vi "Quadrature-Input.vi"() -> ()   [LabVIEW 2020]
panel:
  out "Direction":string
  out "Error String":string
  out "error out":errorcluster
  in  "error in (no error)":errorcluster
  out "ConnectionType Out":i32
  out "DeviceType Out":i32
  in  "Identifier":string="LJM_idANY"
  in  "Connection Type":string="LJM_ctANY"
  in  "Device Type":string="LJM_dtANY"
  out "Revolutions":i32
  in  "?":bool
  in  "Phase Pairs":T1(ring)=enum."T7/T4: FIO6 + FIO7"
  in  "Encoder counts per revolution":i32=400
  in  "stop":bool
  out "Guage":dbl(knob) min=0.0 max=360.0 step=15.0 scale=0.0..360.0
  out "Degrees From Zero":i32
  out "Enc 2's Comp":dbl
  out "Enc Float":dbl
  # "T4 Capable DIO: DIO4, DIO5, DIO6, DIO7, DIO8, DIO9 (aka FIO4, FIO5, FIO6, FIO7, EIO0, EIO1)\n \nT7 Capable DIO: DIO0, DIO1, DIO2, DIO3, DIO6, DIO7 (aka FIO0, FIO1, FIO2, FIO3, FIO6, FIO7)\n\nThe channels must be used in one of the consecutive pairs that can be selected below in \"Phase Pairs\" .The even channel is Phase A and odd channel is Phase B of the encoder.\n\nMake sure to set how many counts per revolution for the encoder."
  # "0"
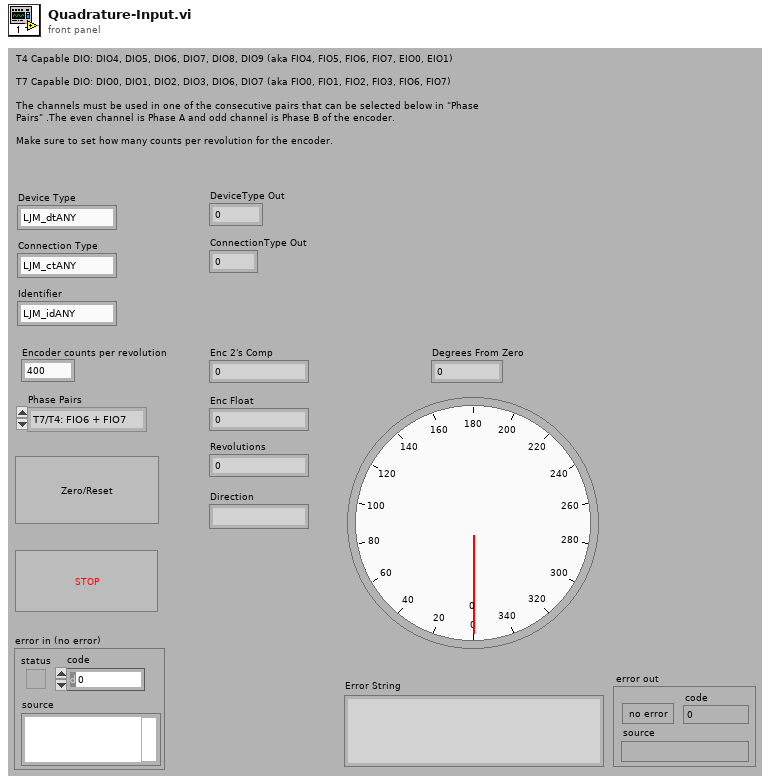
[diagram p1: front panel]
types:
  T1 = enum16{"T7: FIO0 + FIO1", "T7: FIO2 + FIO3", "T7/T4: FIO6 + FIO7", "T4: FIO4 + FIO5", "T4: EIO0 + EIO1"}
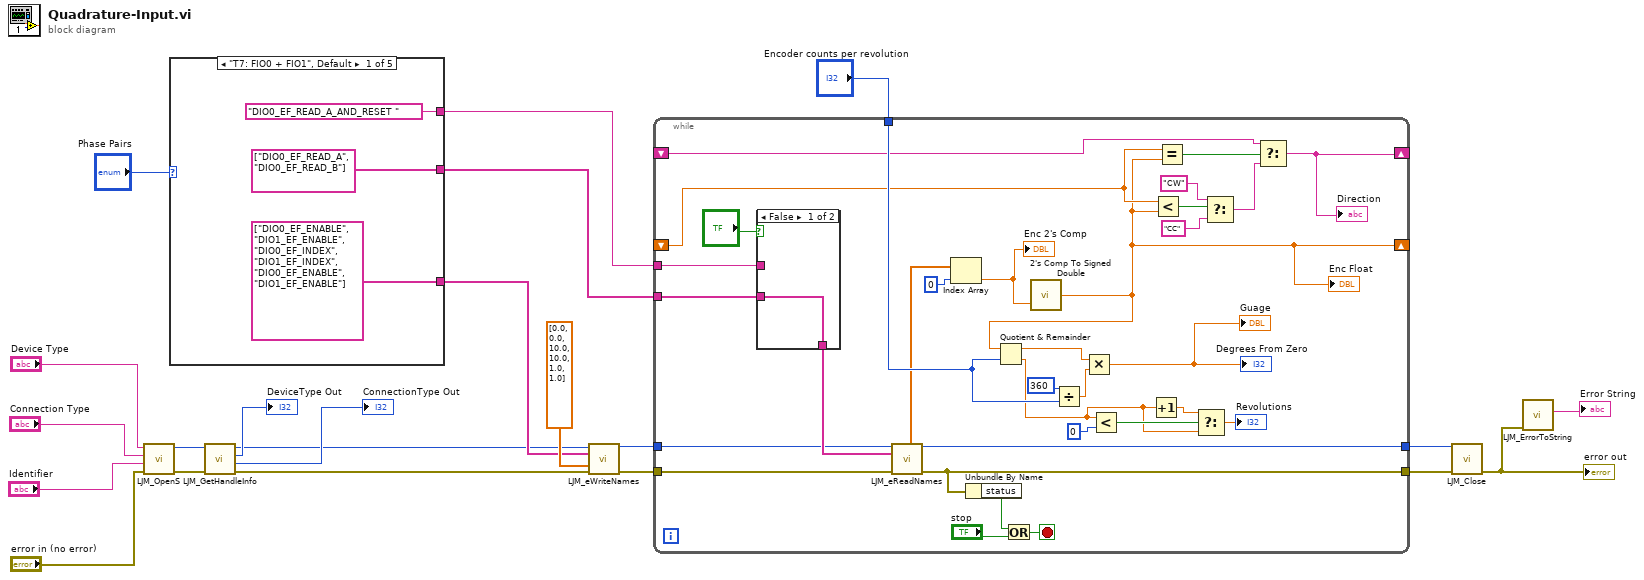
[diagram p0: block diagram]
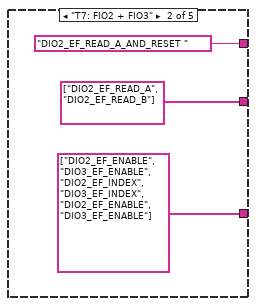
[diagram p2: hidden frame]
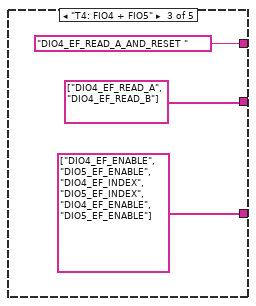
[diagram p3: hidden frame]
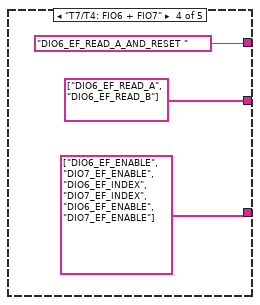
[diagram p4: hidden frame]
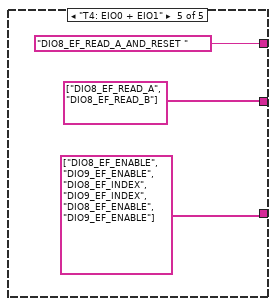
[diagram p5: hidden frame]
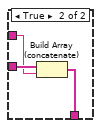
[diagram p6: hidden frame]
diagram:
  n1 = call "LJM_OpenS.vi"("error in"="error in (no error)", "Identifier"="Identifier", "ConnectionType"="Connection Type", "DeviceType"="Device Type") -> ("error out"=w21:errorcluster, "Handle"=w20:i32)  [unwired: 6 in]
  n2 = case shown="\"T7: FIO0 + FIO1\", Default" "Phase Pairs" {
    tunnel: [string[] ["DIO0_EF_READ_A", "DIO0_EF_READ_B"] string[] ["DIO2_EF_READ_A", "DIO2_EF_READ_B"] string[] ["DIO4_EF_READ_A", "DIO4_EF_READ_B"] string[] ["DIO6_EF_READ_A", "DIO6_EF_READ_B"] string[] ["DIO8_EF_READ_A", "DIO8_EF_READ_B"]] -> w9
    tunnel: [string[] ["DIO0_EF_ENABLE", "DIO1_EF_ENABLE", "DIO0_EF_INDEX", "DIO1_EF_INDEX", "DIO0_EF_ENABLE", "DIO1_EF_ENABLE"] string[] ["DIO2_EF_ENABLE", "DIO3_EF_ENABLE", "DIO2_EF_INDEX", "DIO3_EF_INDEX", "DIO2_EF_ENABLE", "DIO3_EF_ENABLE"] string[] ["DIO4_EF_ENABLE", "DIO5_EF_ENABLE", "DIO4_EF_INDEX", "DIO5_EF_INDEX", "DIO4_EF_ENABLE", "DIO5_EF_ENABLE"] string[] ["DIO6_EF_ENABLE", "DIO7_EF_ENABLE", "DIO6_EF_INDEX", "DIO7_EF_INDEX", "DIO6_EF_ENABLE", "DIO7_EF_ENABLE"] string[] ["DIO8_EF_ENABLE", "DIO9_EF_ENABLE", "DIO8_EF_INDEX", "DIO9_EF_INDEX", "DIO8_EF_ENABLE", "DIO9_EF_ENABLE"]] -> w10
    tunnel: ["DIO0_EF_READ_A_AND_RESET " "DIO2_EF_READ_A_AND_RESET " "DIO4_EF_READ_A_AND_RESET " "DIO6_EF_READ_A_AND_RESET " "DIO8_EF_READ_A_AND_RESET "] -> w8
    frame "T7: FIO0 + FIO1", Default {
    }
    frame "T7: FIO2 + FIO3" {
    }
    frame "T4: FIO4 + FIO5" {
    }
    frame "T7/T4: FIO6 + FIO7" {
    }
    frame "T4: EIO0 + EIO1" {
    }
  }
  n3 = call "LJM_GetHandleInfo.vi"("error in"=w21, "Handle In"=w20) -> ("error out"=w13:errorcluster, "ConnectionType"=→"ConnectionType Out":i32, "DeviceType"=→"DeviceType Out":i32, "Handle Out"=w1:i32)  [unwired: 2 in, 4 out]
  n4 = call "LJM_eWriteNames.vi"("Handle In"=w1, "aNames"=w10, "aValuesIn"=dbl[] [0.0, 0.0, 10.0, 10.0, 1.0, 1.0], "error in"=w13) -> ("Handle Out"=w19:i32, "error out"=w18:errorcluster)  [unwired: 9 in, 1 out]
  n5 = while {
    tunnel: w18 -> [w46]
    tunnel: [w67] -> w2
    tunnel: w19 -> [w47]
    tunnel: [w66] -> w3
    tunnel: "Encoder counts per revolution" -> [w64]
    tunnel: w9 -> [w59]
    tunnel: w8 -> [w60]
    shift-right: [w44] -> _
    shift-left: _ -> [w54]
    shift-right: [w49] -> _
    shift-left: _ -> [w50]
    stop <- w70 stop-if-true
    n6 = case shown="False" "?" {
      tunnel: w60 -> [_ w73]
      tunnel: w59 -> [w71 w74]
      tunnel: [w71 w72] -> w58
      frame False {
      }
      frame True {
        n7 = Build Array (concatenate)(w74, w73) -> (w72:string[])
      }
    }
    n8 = call "LJM_eReadNames.vi"("Handle In"=w47, "aNames"=w58, "error in"=w46) -> ("Handle Out"=w66:i32, "aValuesOut"=w63:dbl[], "error out"=w67:errorcluster)  [unwired: 9 in, 1 out]
    n9 = Index Array(array=w63, index=0) -> (element=w45:dbl)
    "Enc 2's Comp" <- w45
    n10 = Unbundle By Name(w67) -> ("status"=w69:bool)
    n11 = Or(x=w69, y="stop") -> (x .or. y?=w70:bool)
    n12 = call "2's Comp To Signed Double.vi"("2's ccomp"=w45) -> ("Signed Double"=w44:dbl)  [unwired: 1 in]
    "Enc Float" <- w44
    n13 = Quotient & Remainder(x=w44, y=w64) -> (x-y*floor(x/y)=w53:dbl, floor(x/y)=w39:dbl)
    n14 = Divide(x=360, y=w64) -> (x/y=w43:dbl)
    n15 = Multiply(x=w53, y=w43) -> (x*y=→"Guage" →"Degrees From Zero":dbl)
    n16 = Less?(x=w39, y=0) -> (x < y?=w40:bool)
    n17 = Increment(x=w39) -> (x+1=w38:dbl)
    n18 = Less?(x=w54, y=w44) -> (x < y?=w56:bool)
    n19 = Equal?(x=w54, y=w44) -> (x = y?=w52:bool)
    n20 = Select(t=w38, s=w40, f=w39) -> (s? t:f=→"Revolutions":dbl)
    n21 = Select(t="CW", s=w56, f="CC") -> (s? t:f=w51:string)
    n22 = Select(t=w50, s=w52, f=w51) -> (s? t:f=w49:string)
    "Direction" <- w49
  }
  n23 = call "LJM_Close.vi"("error in"=w2, "Handle"=w3) -> ("error out"=w6:errorcluster)  [unwired: 9 in]
  "error out" <- w6
  n24 = call "LJM_ErrorToString.vi"("error in"=w6) -> ("String"=→"Error String":string)  [unwired: 10 in]
